vi "IX81 Test Panel.vi"() -> ()   [LabVIEW 2020]
uses:
  <vilib>/Instr/_visa.llb/VISA Configure Serial Port (Instr).vi
panel:
  out "Cmd Success":bool
  out "Objective Z":string
  out "Connected":bool
  out "Waiting for Reply":bool
  out "Last Error":errorcluster
  out "Command History":string
  out "Reply":string
  in  "Command":string
  in  "Quit":bool
  in  "COM Port":refnum<visa-resource-name>="COM4"
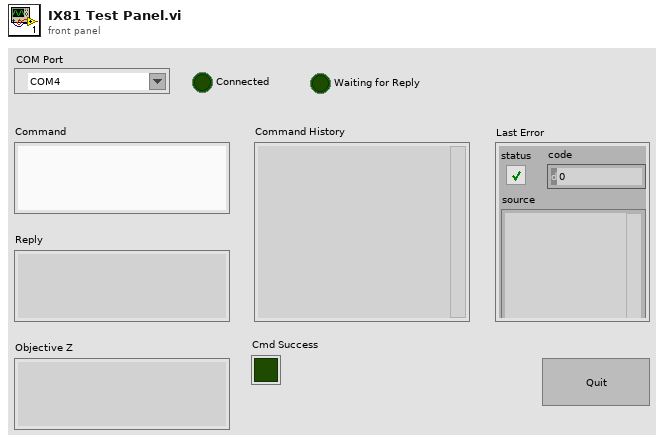
[diagram p1: front panel]
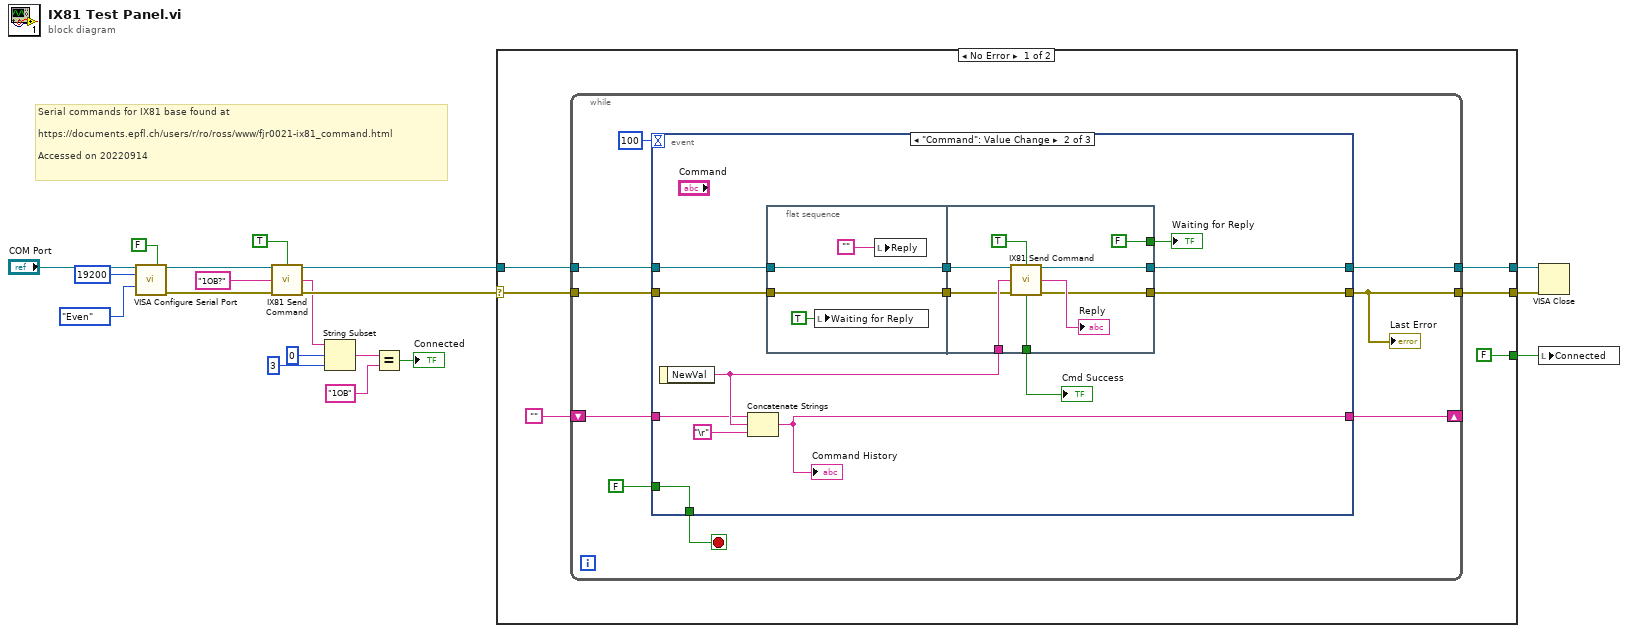
[diagram p0: block diagram]
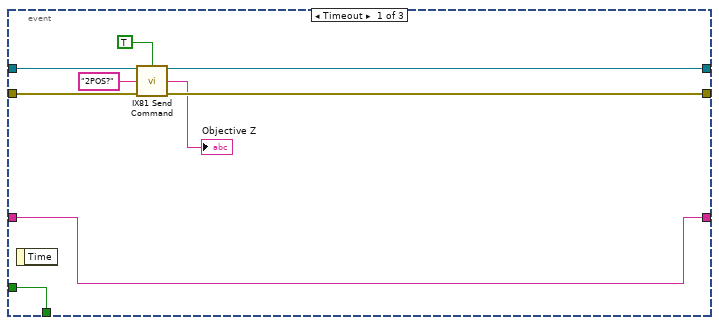
[diagram p2: hidden frame]
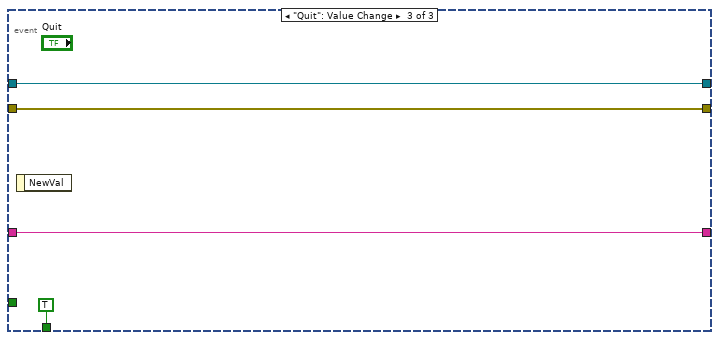
[diagram p3: hidden frame]
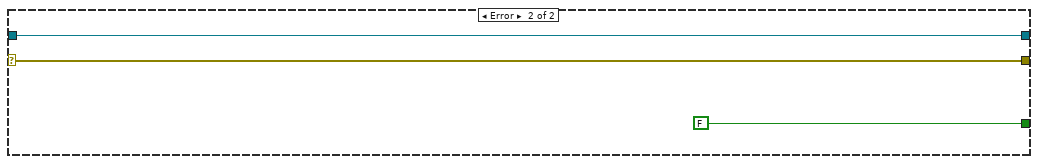
[diagram p4: hidden frame]
diagram:
  # "Serial commands for IX81 base found at\n\nhttps://documents.epfl.ch/users/r/ro/ross/www/fjr0021-ix81_command.html\n\nAccessed on 20220914"
  n1 = call-poly "VISA Configure Serial Port"("VISA resource name"="COM Port", "Enable Termination\nChar (T)"=FALSE ("Enable Termination\nChar (T)"), "baud rate (9600)"=u32 19200, "parity (0:none)"=enum16{"None", "Odd", "Even", "Mark", "Space"}."Even") -> ("VISA resource name out"=w11:refnum<visa-resource-name>, "error out"=w12:errorcluster)  [unwired: 10 in]
  n2 = call "IX81 Send Command.vi"("VISA Ref"=w11, "Wait for Reply (T)"=TRUE, "Command"="1OB?", "Error In"=w12) -> ("VISA Ref Dup"=w9:refnum<visa-resource-name>, "Reply"=w7:string, "Error Out"=w8:errorcluster)  [unwired: 8 in, 1 out]
  n3 = String Subset(string=w7, offset (0)=0, length (rest)=3 ("length (rest)")) -> (substring=w4:string)
  n4 = Equal?(x=w4, y="1OB") -> (x = y?=→"Connected":bool)
  n5 = case shown="No Error" w8 {
    selector: w8 -> [w24 w75]
    tunnel: w9 -> [w25 w76]
    tunnel: [w23 w76] -> w17
    tunnel: [w22 w75] -> w16
    tunnel: [FALSE FALSE] -> w15
    frame No Error {
      n6 = while {
        tunnel: w25 -> [w32]
        tunnel: w24 -> [w31]
        tunnel: [w30] -> w23
        tunnel: [w27] -> w22
        shift-right: [w28] -> _
        shift-left: "" -> [w29]
        stop <- w33 stop-if-true
        n7 = event shown="[1] \"Command\": Value Change" {
          selector: _ -> [_ _ _]
          dyn-events: _ -> [_ _ _]
          timeout: 100 -> [_ _ _]
          tunnel: FALSE -> [w43 w56 _]
          tunnel: [w43 w56 TRUE] -> w33
          tunnel: w32 -> [w41 w55 w73]
          tunnel: w31 -> [w40 w54 w72]
          tunnel: [w37 w50 w73] -> w30
          tunnel: [w36 w51 w72] -> w27
          tunnel: w29 -> [w42 w47 w70]
          tunnel: [w42 w46 w70] -> w28
          event Timeout {
            n8 = event-data() -> ()  [unwired: 1 in, 1 out]
            n9 = call "IX81 Send Command.vi"("VISA Ref"=w41, "Wait for Reply (T)"=TRUE, "Command"="2POS?", "Error In"=w40) -> ("VISA Ref Dup"=w37:refnum<visa-resource-name>, "Reply"=→"Objective Z":string, "Error Out"=w36:errorcluster)  [unwired: 8 in, 1 out]
          }
          event "Command": Value Change {
            n10 = event-data() -> ("NewVal"=w49:string)  [unwired: 1 in]
            n11 = Concatenate Strings(w47, w49, "\r") -> (w46:string)
            "Command History" <- w46
            n12 = flat-sequence {
              tunnel: w54 -> [w59]
              tunnel: w55 -> [w60]
              tunnel: [w60] -> w53
              tunnel: [w59] -> w52
              tunnel: w49 -> [w68]
              tunnel: w53 -> [w69]
              tunnel: w52 -> [w67]
              tunnel: [w65] -> w51
              tunnel: [w64] -> w50
              tunnel: [FALSE] -> w45
              tunnel: [w61] -> w44
              frame #0 {
                n13 = local write "Waiting for Reply"(TRUE ("Waiting for Cmd")) -> ()
                n14 = local write "Reply"("") -> ()
              }
              frame #1 {
                n15 = call "IX81 Send Command.vi"("VISA Ref"=w69, "Wait for Reply (T)"=TRUE, "Command"=w68, "Error In"=w67) -> ("VISA Ref Dup"=w64:refnum<visa-resource-name>, "Reply"=→"Reply":string, "Cmd Success"=w61:bool, "Error Out"=w65:errorcluster)  [unwired: 8 in]
              }
            }
            "Waiting for Reply" <- w45
            "Cmd Success" <- w44
          }
          event "Quit": Value Change {
            n16 = event-data() -> ()  [unwired: 1 in, 1 out]
          }
        }
        "Last Error" <- w27
      }
    }
    frame Error {
    }
  }
  n17 = VISA Close(VISA resource name=w17, error in (no error)=w16) -> ()  [unwired: 1 out]
  n18 = local write "Connected"(w15) -> ()
